vi "Voltage Logging.vi"() -> ()   [LabVIEW 2014]
uses:
  States.ctl
  <vilib>/Utility/miscctls.llb/LVForegroundBackgroundColorsTypeDef.ctl
  <vilib>/DAQmx/read.llb/DAQmx Read (Analog 1D Wfm NChan 1Samp).vi
  <vilib>/DAQmx/miscellaneous.llb/DAQmx Fill In Error Info.vi
  <vilib>/DAQmx/create/channels.llb/DAQmx Create Channel (AI-Voltage-Basic).vi
panel:
  out "Timer":dbl format="%#_g sec"
  in  "maximum value":dbl=1.0 format="%#_13g"
  in  "minimum value":dbl=-1.0 format="%#_13g"
  in  "input terminal configuration":i32(ring)=10083 items=["default"=-1, "RSE"=10083, "NRSE"=10078, "Differential"=10106, "Pseudodifferential"=12529]
  in  "Connect":bool
  out "Logging speed calculated":dbl=3.6
  in  "Time format":bool=TRUE
  out "Error messeage":string
  out "Communication with CDaq":bool
  in  "Channels":tag="cDAQ3Mod1/ai0:7, cDAQ3Mod2/ai0:7, cDAQ3Mod3/ai0:7"
  in  "Upper Limit 3":dbl[](array[numeric])=[0.0, 0.0, 0.0, 0.0, 0.0, 0.0, 0.0, 0.0, 1000.0, 1000.0, 1000.0, 1000.0, 1000.0, 1000.0, 1000.0, 1000.0, 1000.0, 1000.0, 1000.0, 1000.0, 1000.0, 1000.0, 1000.0, 1000.0, 1000.0, 1000.0, 1000.0, 1000.0, 1000.0, 1000.0, 1000.0, 1000.0]
  in  "Upper Limit 2":dbl[](array[numeric])=[0.0, 0.0, 0.0, 0.0, 0.0, 0.0, 0.0, 0.0, 1000.0, 1000.0, 1000.0, 1000.0, 1000.0, 1000.0, 1000.0, 1000.0, 1000.0, 1000.0, 1000.0, 1000.0, 1000.0, 1000.0, 1000.0, 1000.0, 1000.0, 1000.0, 1000.0, 1000.0, 1000.0, 1000.0, 1000.0, 1000.0]
  in  "Lower Limit 3":dbl[](array[numeric])=[-400.0, -400.0, -400.0, -400.0, -400.0, -400.0, -400.0, -400.0, -1000.0, -1000.0, -1000.0, -1000.0, -1000.0, -1000.0, -1000.0, -1000.0, -1000.0, -1000.0, -1000.0, -1000.0, -1000.0, -1000.0, -1000.0, -1000.0, -1000.0, -1000.0, -1000.0, -1000.0, -1000.0, -1000.0, -1000.0, -1000.0, -10000.0, -1000.0]
  in  "Lower Limit 2":dbl[](array[numeric])=[-400.0, -400.0, -400.0, -400.0, -400.0, -400.0, -400.0, -400.0, -1000.0, -1000.0, -1000.0, -1000.0, -1000.0, -1000.0, -1000.0, -1000.0, -1000.0, -1000.0, -1000.0, -1000.0, -1000.0, -1000.0, -1000.0, -1000.0, -1000.0, -1000.0, -1000.0, -1000.0, -1000.0, -1000.0, -1000.0, -1000.0, -10000.0, -1000.0]
  in  "Channel Name 3":string[](array[string])=["STDFA-13", "STDFA-14", "STDFA-15", "STDFA-16", "STDFA-17", "STDFA-18", "No", "No", "Sample 2-1", "Sample 2-2", "Sample 2-3", "Sample 2-4", "Sample 2-5", "Sample 2-6", "Sample 2-7", "Sample 2-8", "Sample 3-1", "Sample 3-2", "Sample 3-3", "Sample 3-4", "Sample 3-5", "Sample 3-6", "Sample 3-7", "Sample 3-8", "Channel 25", "Channel 26", "Channel 27", "Channel 28", "Channel 29", "Channel 30", "Channel 31", "Channel 32"]
  in  "Channel Name 2":string[](array[string])=["IND-7", "IND-8", "IND-9", "IND-10", "IND-11", "IND-12", "No", "No", "Sample 2-1", "Sample 2-2", "Sample 2-3", "Sample 2-4", "Sample 2-5", "Sample 2-6", "Sample 2-7", "Sample 2-8", "Sample 3-1", "Sample 3-2", "Sample 3-3", "Sample 3-4", "Sample 3-5", "Sample 3-6", "Sample 3-7", "Sample 3-8", "Channel 25", "Channel 26", "Channel 27", "Channel 28", "Channel 29", "Channel 30", "Channel 31", "Channel 32"]
  out "To Chart":dbl[](array[numeric])=[70.54695373277418, 10.349711390143883, 7.51922355130685, 18.709524383023034, 7.8154373944745705, 12.02825650884127, -6.402827028058501, -31.548091462286674, -93.31739444104286, 3.5496163088758026, 6.22112697925856, 6.715851179669773, 4.506083089902143, 6.484979886054426, 3.747505987517876, -20.0652183361864, -91.63029877543632, -0.5237737702217623, 6.226074724835393, 9.419905426557538, -0.9188868578980165, 8.59675318650909, 7.740674854943624, -15.27466285302956]
  out "Stop":bool=TRUE
  out "In Range?  4":bool[](array[boolean])=[TRUE, TRUE, TRUE, TRUE, TRUE, TRUE, TRUE, TRUE]
  out "In Range?  3":bool[](array[boolean])=[TRUE, TRUE, TRUE, TRUE, TRUE, TRUE, TRUE, TRUE]
  out "In Range?  2":bool[](array[boolean])=[TRUE, TRUE, TRUE, TRUE, TRUE, TRUE, TRUE, TRUE]
  out "SAMPLE 3":dbl[](array[numeric])=[-91.63029877543632, -0.5237737702217623, 6.226074724835393, 9.419905426557538, -0.9188868578980165, 8.59675318650909, 7.740674854943624, -15.27466285302956] format="%#.1f"
  out "SAMPLE 2":dbl[](array[numeric])=[-93.31739444104286, 3.5496163088758026, 6.22112697925856, 6.715851179669773, 4.506083089902143, 6.484979886054426, 3.747505987517876, -20.0652183361864] format="%#.1f"
  out "SAMPLE 1":dbl[](array[numeric])=[70.54695373277418, 10.349711390143883, 7.51922355130685, 18.709524383023034, 7.8154373944745705, 12.02825650884127, -6.402827028058501, -31.548091462286674] format="%#.1f"
  out "CHANNEL 1-8 SAMPLE 3":T1(graph)={"Numeric"=-91.56444653578738, "Numeric"=-0.2932911360215918, "Numeric"=6.489483443591846, "Numeric"=9.716240232547184, "Numeric"=-0.6554781327134408, "Numeric"=8.761383634660817, "Numeric"=7.740674854943624, "Numeric"=-15.406367224861299}
  out "CHANNEL 1-8   SAMPLE 2":T1(graph)={"Numeric"=-92.75670672596173, "Numeric"=3.945395666258387, "Numeric"=6.682869566286414, "Numeric"=6.913740860038615, "Numeric"=4.60502792945394, "Numeric"=6.419016659336254, "Numeric"=3.7145243744040615, "Numeric"=-20.16416317419381}
  in  "Channel Name":string[](array[string])=["LKS-1", "LKS-2", "LKS-3", "LKS-4", "LKS-5", "LKS-6", "No", "No", "Sample 2-1", "Sample 2-2", "Sample 2-3", "Sample 2-4", "Sample 2-5", "Sample 2-6", "Sample 2-7", "Sample 2-8", "Sample 3-1", "Sample 3-2", "Sample 3-3", "Sample 3-4", "Sample 3-5", "Sample 3-6", "Sample 3-7", "Sample 3-8", "Channel 25", "Channel 26", "Channel 27", "Channel 28", "Channel 29", "Channel 30", "Channel 31", "Channel 32"]
  in  "Logging Speed":dbl=0.001 format="%#_g h"
  out "CHANNEL 1-8 SAMPLE 1":T1(graph)={"Numeric"=69.98743853157956, "Numeric"=9.888934299429126, "Numeric"=7.025533812893019, "Numeric"=18.347485234778834, "Numeric"=7.617961499019248, "Numeric"=11.929518560566871, "Numeric"=-6.43573967719425, "Numeric"=-31.44935350980207}
  in  "Lower Limit":dbl[](array[numeric])=[-400.0, -400.0, -400.0, -400.0, -400.0, -400.0, -400.0, -400.0, -1000.0, -1000.0, -1000.0, -1000.0, -1000.0, -1000.0, -1000.0, -1000.0, -1000.0, -1000.0, -1000.0, -1000.0, -1000.0, -1000.0, -1000.0, -1000.0, -1000.0, -1000.0, -1000.0, -1000.0, -1000.0, -1000.0, -1000.0, -1000.0, -10000.0, -1000.0]
  in  "Upper Limit":dbl[](array[numeric])=[0.0, 0.0, 0.0, 0.0, 0.0, 0.0, 0.0, 0.0, 1000.0, 1000.0, 1000.0, 1000.0, 1000.0, 1000.0, 1000.0, 1000.0, 1000.0, 1000.0, 1000.0, 1000.0, 1000.0, 1000.0, 1000.0, 1000.0, 1000.0, 1000.0, 1000.0, 1000.0, 1000.0, 1000.0, 1000.0, 1000.0]
  out "Potential (mV)":dbl[](array[numeric])=[70.54695373277418, 10.349711390143883, 7.51922355130685, 18.709524383023034, 7.8154373944745705, 12.02825650884127, -6.402827028058501, -31.548091462286674, -93.31739444104286, 3.5496163088758026, 6.22112697925856, 6.715851179669773, 4.506083089902143, 6.484979886054426, 3.747505987517876, -20.0652183361864, -91.63029877543632, -0.5237737702217623, 6.226074724835393, 9.419905426557538, -0.9188868578980165, 8.59675318650909, 7.740674854943624, -15.27466285302956] format="%#.1f"
  in  "Start":bool
  in  "Stop":bool
  # "Potential Logging 2015"
  # "Time until next logging point"
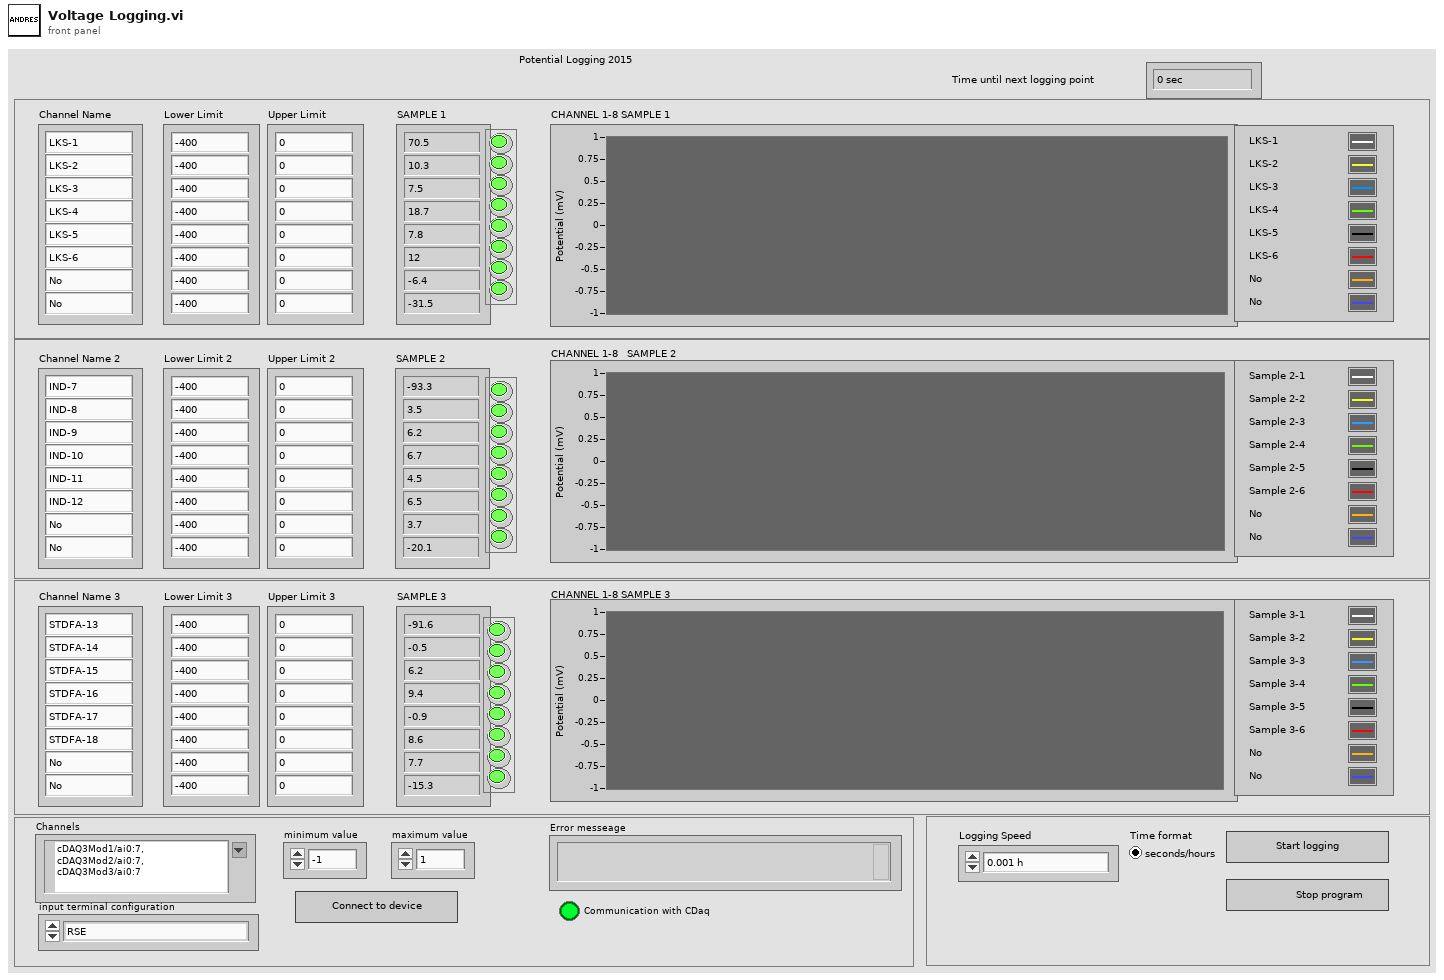
[diagram p1: front panel]
types:
  T1 = cluster{"Numeric":dbl, "Numeric":dbl, "Numeric":dbl, "Numeric":dbl, "Numeric":dbl, "Numeric":dbl, "Numeric":dbl, "Numeric":dbl}
  T2 = typedef "LVForegroundBackgroundColorsTypeDef.ctl" = cluster{"Foreground Color":u32, "Background Color":u32}
  T3 = enum8{"Enabled", "Disabled", "Disabled and Grayed Out"}
  T4 = typedef "States.ctl" = enum16{"Init", "Create File", "Logging", "Stop Program", "Connect"}
  T5 = enum16{"open", "replace", "create", "open or create", "replace or create", "replace or create with confirmation"}
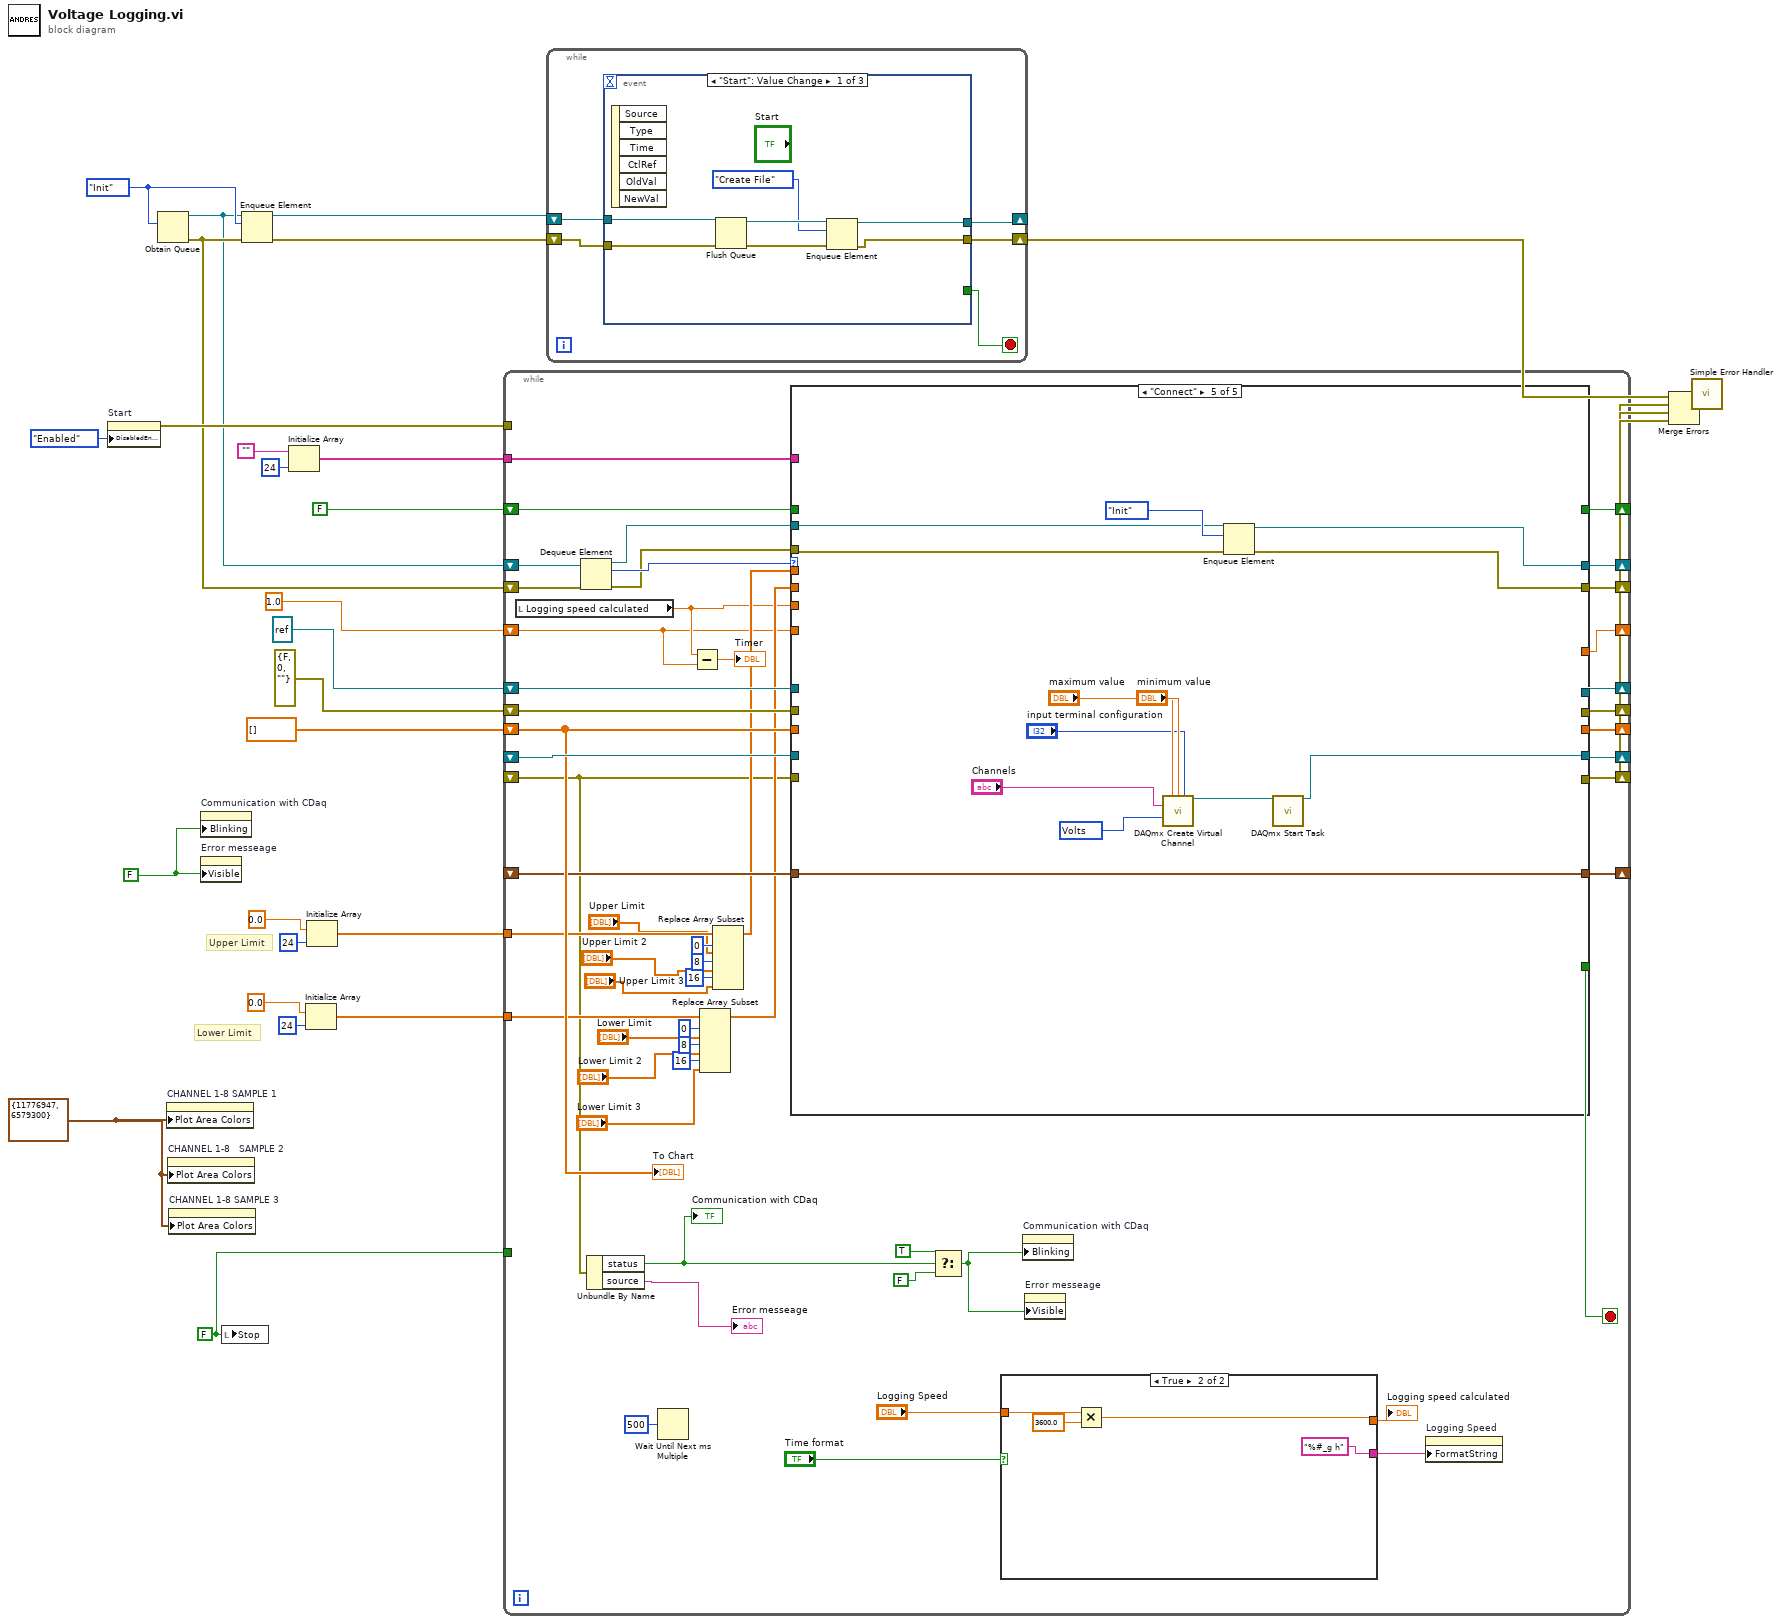
[diagram p0: block diagram]
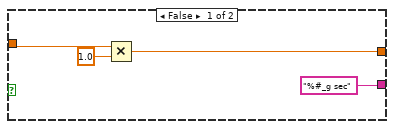
[diagram p2: hidden frame]
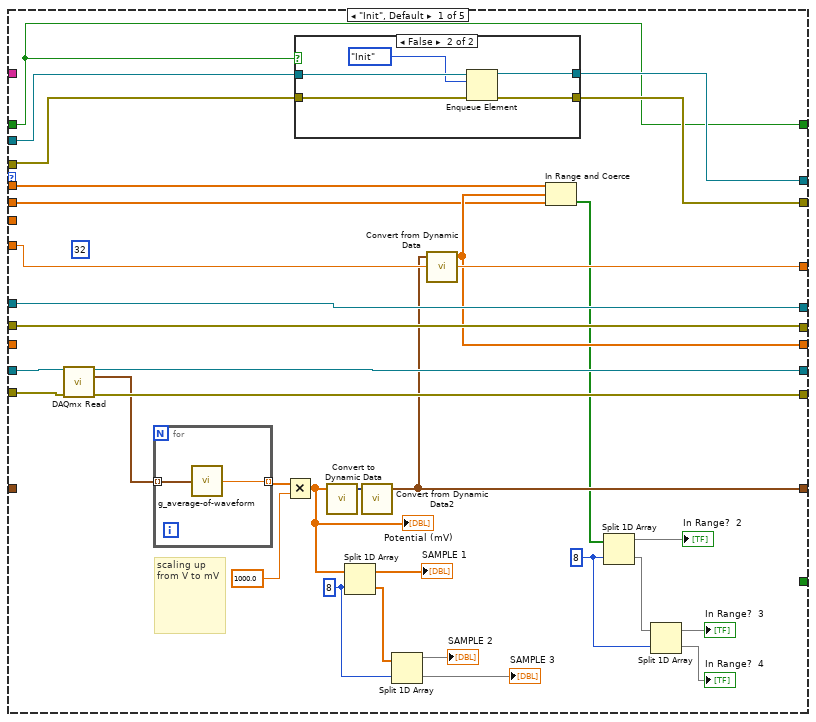
[diagram p3: hidden frame]
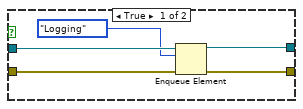
[diagram p4: hidden frame]
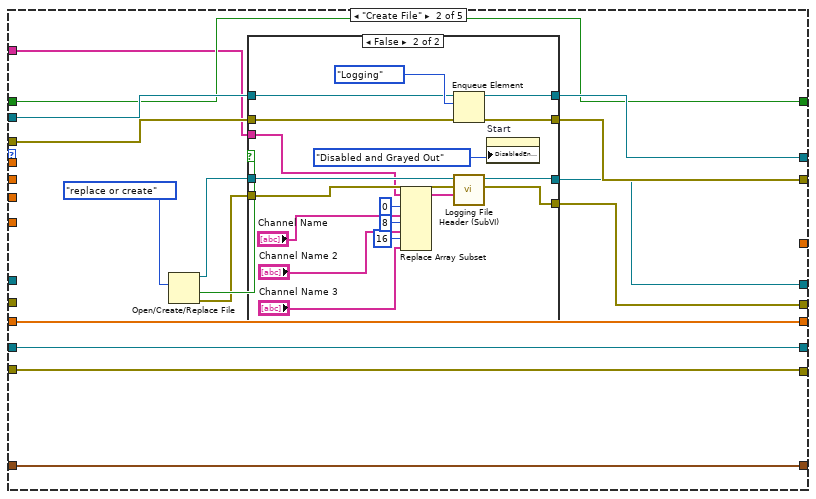
[diagram p5: hidden frame]
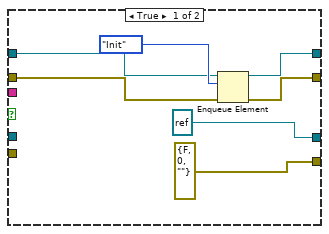
[diagram p6: hidden frame]
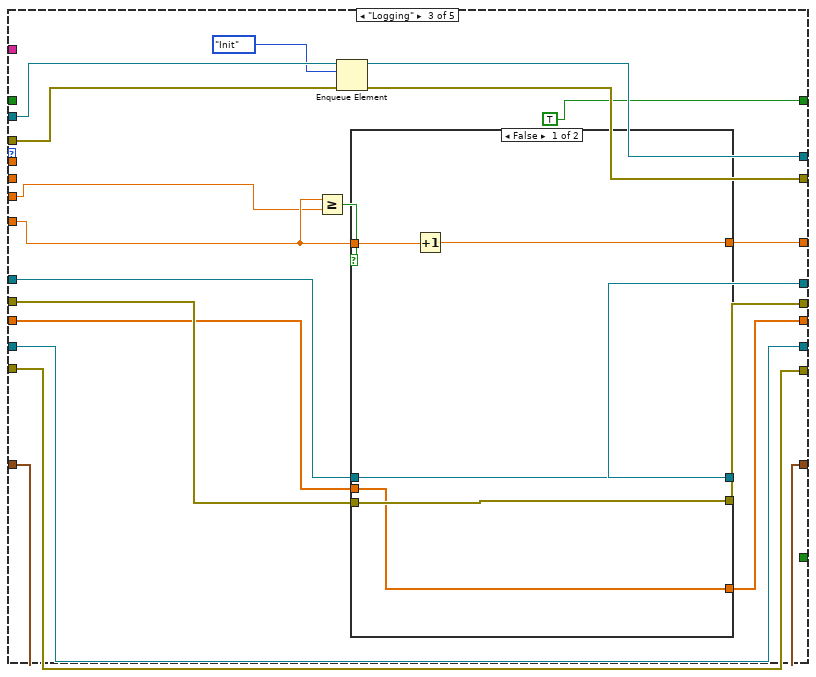
[diagram p7: hidden frame]
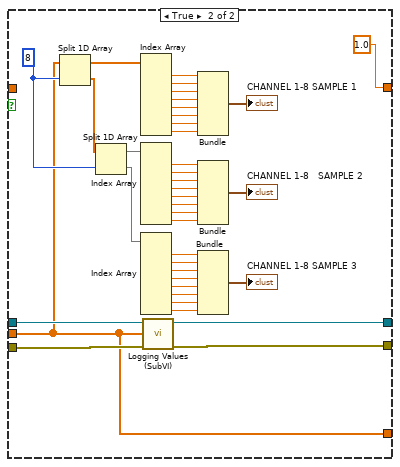
[diagram p8: hidden frame]
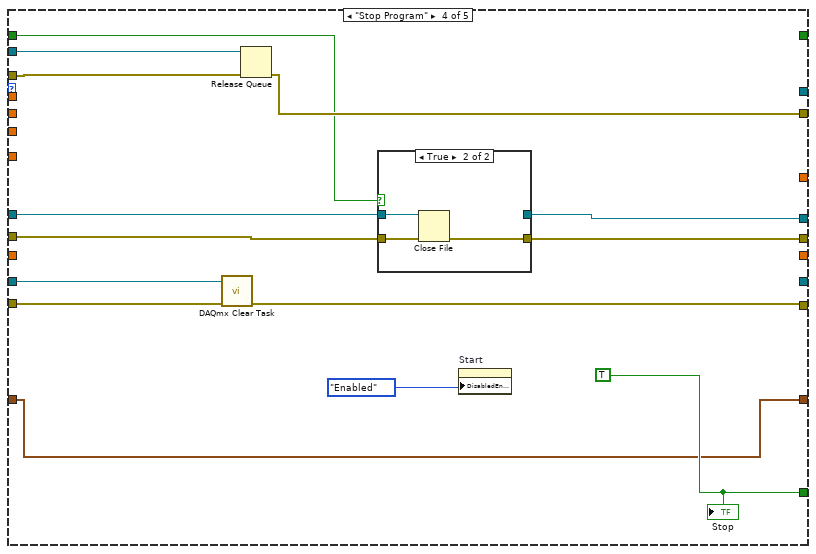
[diagram p9: hidden frame]
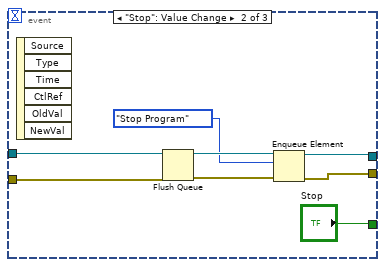
[diagram p11: hidden frame]
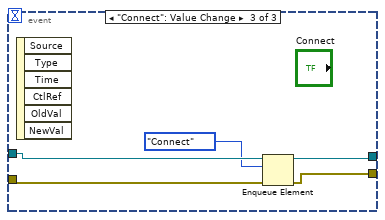
[diagram p12: hidden frame]
diagram:
  w1 = FALSE ("Visible")
  w11 = FALSE ("Stop")
  w12 = T2 {"Foreground Color"=11776947, "Background Color"=6579300} ("Plot Area:Colors 2")
  w27 = States."Init" ("States")
  # "Lower Limit"
  # "Upper Limit"
  n1 = property on="Start" class="Bool"("DisabledEnum"=T3."Enabled" ("Disabled")) -> (error out=w22:errorcluster)  [unwired: 2 in, 1 out]
  n2 = Obtain Queue(element data type=w27) -> (queue out=w19:refnum<queue>, error out=w20:errorcluster)  [unwired: 4 in, 1 out]
  n3 = property on="CHANNEL 1-8 SAMPLE 1" class="WFChart (strict)"("Plot Area Colors"=w12) -> ()  [unwired: 2 in, 2 out]
  n4 = property on="CHANNEL 1-8   SAMPLE 2" class="WFChart (strict)"("Plot Area Colors"=w12) -> ()  [unwired: 2 in, 2 out]
  n5 = property on="CHANNEL 1-8 SAMPLE 3" class="WFChart (strict)"("Plot Area Colors"=w12) -> ()  [unwired: 2 in, 2 out]
  n6 = property on="Communication with CDaq" class="Bool (strict)"("Blinking"=w1) -> ()  [unwired: 2 in, 2 out]
  n7 = property on="Error messeage" class="Str"("Visible"=w1) -> ()  [unwired: 2 in, 2 out]
  n8 = local write "Stop"(w11) -> ()
  n9 = Enqueue Element(queue=w19, element=w27, error in (no error)=w20) -> (queue out=w29:refnum<queue>, error out=w28:errorcluster)  [unwired: 1 in, 1 out]
  n10 = Initialize Array("", 24 ("dimension size")) -> (w8:string[])
  n11 = Initialize Array(0.0, 24 ("dimension size")) -> (w2:dbl[])
  n12 = Initialize Array(0.0, 24 ("dimension size")) -> (w3:dbl[])
  n13 = while {
    shift-right: [w77] -> _
    shift-left: w19 -> [w81]
    shift-right: [w76] -> w13
    shift-left: w20 -> [w82]
    shift-right: [w74] -> w15
    shift-left: _ -> [w42]
    shift-right: [w72] -> _
    shift-left: _ -> [w73]
    shift-right: [w63] -> _
    shift-left: dbl[] [] ("Array") -> [w61]
    shift-right: [w70] -> _
    shift-left: refnum<file> refnum ("refnum out") -> [w71]
    shift-right: [w69] -> w14
    shift-left: errorcluster {"status"=FALSE, "code"=0, "source"=""} ("error out") -> [w68]
    shift-right: [w66] -> _
    shift-left: FALSE -> [w67]
    shift-right: [w64] -> _
    shift-left: 1.0 -> [w31]
    tunnel: w22 -> [_]
    shift-right: [w62] -> _
    shift-left: _ -> [w60]
    tunnel: w11 -> [_]
    tunnel: w8 -> [w59]
    tunnel: w3 -> [w52]
    tunnel: w2 -> [w50]
    stop <- w75 stop-if-true
    n14 = local read "Logging speed calculated"() -> (w32:dbl)
    n15 = Dequeue Element(queue=w81, error in (no error)=w82) -> (queue out=w79:refnum<queue>, element=w80:T4, error out=w78:errorcluster)  [unwired: 1 in, 1 out]
    n16 = Unbundle By Name(w42) -> ("status"=w40:bool, "source"=→"Error messeage":string)
    "Communication with CDaq" <- w40
    n17 = Wait Until Next ms Multiple(millisecond multiple=u32 500) -> ()  [unwired: 1 out]
    n18 = Subtract(x=w32, y=w31) -> (x-y=→"Timer":dbl)
    n19 = Replace Array Subset(array=w50, new element #1="Lower Limit", index #1=0 ("index"), new element #2="Lower Limit 2", index #2=8 ("index"), new element #3="Lower Limit 3", index #3=16 ("index")) -> (w49:dbl[])
    n20 = Replace Array Subset(array=w52, new element #1="Upper Limit", index #1=0 ("index"), new element #2="Upper Limit 2", index #2=8 ("index"), new element #3="Upper Limit 3", index #3=16 ("index")) -> (w51:dbl[])
    n21 = case shown="\"Connect\"" w80 {
      tunnel: w79 -> [w122 w150 w194 w247 w268]
      tunnel: w78 -> [w111 w149 w193 w246 w266]
      tunnel: [w121 w148 w192 _ w267] -> w77
      tunnel: [w120 w147 w191 w245 w265] -> w76
      tunnel: [_ _ _ w242 _] -> w75
      tunnel: w42 -> [w119 w143 w178 w250 _]
      tunnel: w73 -> [w118 w144 w177 w251 _]
      tunnel: [w116 w143 w178 w243 _] -> w74
      tunnel: [w117 w144 w177 _ w258] -> w72
      tunnel: [w106 w145 w180 _ _] -> w63
      tunnel: w61 -> [_ w145 w181 _ _]
      tunnel: w71 -> [w114 _ w186 w249 _]
      tunnel: [w114 w138 w189 w241 _] -> w70
      tunnel: [w113 w137 w188 w244 _] -> w69
      tunnel: w68 -> [w113 _ w185 w248 _]
      tunnel: w67 -> [w115 w142 _ w240 _]
      tunnel: [w115 w142 TRUE _ _] -> w66
      tunnel: w31 -> [w112 _ w182 _ _]
      tunnel: [w112 _ w184 _ _] -> w64
      tunnel: [w105 w136 w179 w238 w257] -> w62
      tunnel: w60 -> [_ w136 w179 w238 w257]
      tunnel: w59 -> [_ w135 _ _ _]
      tunnel: w51 -> [w92 _ _ _ _]
      tunnel: w49 -> [w91 _ _ _ _]
      tunnel: w32 -> [_ _ w176 _ _]
      frame "Init", Default {
        w96 = 8 ("index")
        w104 = 8 ("index")
        (unwired) 32 ("index")
        # "scaling up from V to mV"
        n22 = call-poly <vilib>:"DAQmx Read.vi"("task/channels in"=w118, "error in"=w119) -> ("task out"=w117:refnum<k21>, "data"=w110:waveform(dbl)[], "error out"=w116:errorcluster)  [unwired: 11 in]
        n23 = for {
          tunnel: w110 -> [w124] mode=indexing
          tunnel: [w123] -> w109 mode=indexing
          n24 = call "g_average-of-waveform.vi"("element"=w124) -> ("array average"=w123:dbl)
        }
        n25 = Multiply(x=w109, y=1000.0) -> (x*y=w102:dbl[])
        "Potential (mV)" <- w102
        n26 = case shown="False" w115 {
          tunnel: w122 -> [w129 w134]
          tunnel: w111 -> [w128 w133]
          tunnel: [w127 w132] -> w121
          tunnel: [w126 w131] -> w120
          frame True {
            n27 = Enqueue Element(queue=w129, element=States."Logging" ("States"), error in (no error)=w128) -> (queue out=w127:refnum<queue>, error out=w126:errorcluster)  [unwired: 1 in, 1 out]
          }
          frame False {
            n28 = Enqueue Element(queue=w134, element=States."Init" ("States"), error in (no error)=w133) -> (queue out=w132:refnum<queue>, error out=w131:errorcluster)  [unwired: 1 in, 1 out]
          }
        }
        n29 = call "Convert to Dynamic Data"("Array"=w102) -> ("Dynamic Data Type"=w107:dynamicdata)  [unwired: 3 in]
        n30 = Split 1D Array(array=w102, index=w104) -> (first subarray=→"SAMPLE 1":dbl[], second subarray=w103:dbl[])
        n31 = call "Convert from Dynamic Data2"("Dynamic Data Type"=w107) -> ("Array of Waveform"=w105:waveform(dbl)[])  [unwired: 3 in]
        n32 = Split 1D Array(array=w103, index=w104) -> (first subarray=→"SAMPLE 2":dbl[], second subarray=→"SAMPLE 3":dbl[])
        n33 = call "Convert from Dynamic Data"("Dynamic Data Type"=w105) -> ("Array"=w106:dbl[])  [unwired: 3 in]
        n34 = In Range and Coerce(upper limit=w92, x=w106, lower limit=w91) -> (In Range?=w97:bool[])  [unwired: 1 out]
        n35 = Split 1D Array(array=w97, index=w96) -> (first subarray=→"In Range?  2":bool[], second subarray=w98:bool[])
        n36 = Split 1D Array(array=w98, index=w96) -> (first subarray=→"In Range?  3":bool[], second subarray=→"In Range?  4":bool[])
      }
      frame "Create File" {
        n37 = Open/Create/Replace File(operation (0:open)=T5."replace or create") -> (refnum out=w140:refnum<file>, cancelled=w141:bool, error out=w139:errorcluster)  [unwired: 5 in]
        n38 = case shown="False" w141 {
          tunnel: w150 -> [w156 w174]
          tunnel: w149 -> [w155 w173]
          tunnel: [w154 w172] -> w148
          tunnel: [w153 w171] -> w147
          tunnel: w140 -> [_ w170]
          tunnel: w139 -> [_ w169]
          tunnel: [refnum<file> refnum ("refnum out") w168] -> w138
          tunnel: [errorcluster {"status"=FALSE, "code"=0, "source"=""} ("error out") w167] -> w137
          tunnel: w135 -> [_ w158]
          frame True {
            n39 = Enqueue Element(queue=w156, element=States."Init" ("States"), error in (no error)=w155) -> (queue out=w154:refnum<queue>, error out=w153:errorcluster)  [unwired: 1 in, 1 out]
          }
          frame False {
            n40 = Replace Array Subset(array=w158, new element #1="Channel Name", index #1=0 ("index"), new element #2="Channel Name 2", index #2=8 ("index"), new element #3="Channel Name 3", index #3=16 ("index")) -> (w159:string[])
            n41 = Enqueue Element(queue=w174, element=States."Logging" ("States"), error in (no error)=w173) -> (queue out=w172:refnum<queue>, error out=w171:errorcluster)  [unwired: 1 in, 1 out]
            n42 = call "Logging File Header (SubVI).vi"("Channel Name"=w159, "error out"=w169, "file (use dialog)"=w170) -> ("error out 2"=w167:errorcluster, "refnum out"=w168:refnum<file>)  [unwired: 7 in]
            n43 = property on="Start" class="Bool"("DisabledEnum"=T3."Disabled and Grayed Out" ("Disabled")) -> ()  [unwired: 2 in, 2 out]
          }
        }
      }
      frame "Logging" {
        n44 = Greater Or Equal?(x=w182, y=w176) -> (x >= y?=w183:bool)
        n45 = Enqueue Element(queue=w194, element=States."Init" ("States"), error in (no error)=w193) -> (queue out=w192:refnum<queue>, error out=w191:errorcluster)  [unwired: 1 in, 1 out]
        n46 = case shown="False" w183 {
          tunnel: [w199 w237] -> w189
          tunnel: [w198 w236] -> w188
          tunnel: w181 -> [w195 w202]
          tunnel: w186 -> [w199 w235]
          tunnel: w185 -> [w198 w234]
          tunnel: w182 -> [w197 _]
          tunnel: [w196 1.0] -> w184
          tunnel: [w195 w202] -> w180
          frame False {
            n47 = Increment(x=w197) -> (x+1=w196:dbl)
          }
          frame True {
            w229 = 8 ("index")
            n48 = Split 1D Array(array=w202, index=w229) -> (first subarray=w226:dbl[], second subarray=w230:dbl[])
            n49 = Split 1D Array(array=w230, index=w229) -> (first subarray=w228:dbl[], second subarray=w227:dbl[])
            n50 = Index Array(array=w226) -> (element #1=w225:dbl, element #2=w224:dbl, element #3=w223:dbl, element #4=w222:dbl, element #5=w221:dbl, element #6=w220:dbl, element #7=w219:dbl, element #8=w218:dbl)  [unwired: 8 in]
            n51 = Index Array(array=w228) -> (element #1=w217:dbl, element #2=w215:dbl, element #3=w214:dbl, element #4=w213:dbl, element #5=w212:dbl, element #6=w211:dbl, element #7=w210:dbl, element #8=w209:dbl)  [unwired: 8 in]
            n52 = Index Array(array=w227) -> (element #1=w216:dbl, element #2=w208:dbl, element #3=w207:dbl, element #4=w206:dbl, element #5=w205:dbl, element #6=w204:dbl, element #7=w203:dbl, element #8=w200:dbl)  [unwired: 8 in]
            n53 = call "Logging Values (SubVI).vi"("error in (no error)"=w234, "Array"=w202, "Byte Stream File in"=w235) -> ("error out"=w236:errorcluster, "Byte Stream File out"=w237:refnum<file>)  [unwired: 7 in]
            n54 = Bundle("Numeric"=w225, "Numeric"=w224, "Numeric"=w223, "Numeric"=w222, "Numeric"=w221, "Numeric"=w220, "Numeric"=w219, "Numeric"=w218) -> (→"CHANNEL 1-8 SAMPLE 1":T1)  [unwired: 1 in]
            n55 = Bundle("Numeric"=w217, "Numeric"=w215, "Numeric"=w214, "Numeric"=w213, "Numeric"=w212, "Numeric"=w211, "Numeric"=w210, "Numeric"=w209) -> (→"CHANNEL 1-8   SAMPLE 2":T1)  [unwired: 1 in]
            n56 = Bundle("Numeric"=w216, "Numeric"=w208, "Numeric"=w207, "Numeric"=w206, "Numeric"=w205, "Numeric"=w204, "Numeric"=w203, "Numeric"=w200) -> (→"CHANNEL 1-8 SAMPLE 3":T1)  [unwired: 1 in]
          }
        }
      }
      frame "Stop Program" {
        w242 = TRUE
        n57 = call <vilib>:"DAQmx Clear Task.vi"("task in"=w251, "error in"=w250) -> ("error out"=w243:errorcluster)  [unwired: 13 in]
        n58 = Release Queue(queue=w247, error in (no error)=w246) -> (error out=w245:errorcluster)  [unwired: 1 in, 2 out]
        n59 = case shown="True" w240 {
          tunnel: w249 -> [w253 w256]
          tunnel: w248 -> [w252 w255]
          tunnel: [w252 w254] -> w244
          tunnel: [w253 _] -> w241
          frame False {
          }
          frame True {
            n60 = Close File(refnum=w256, error in=w255) -> (error out=w254:errorcluster)  [unwired: 1 out]
          }
        }
        n61 = property on="Start" class="Bool"("DisabledEnum"=T3."Enabled" ("Disabled")) -> ()  [unwired: 2 in, 2 out]
        "Stop" <- w242
      }
      frame "Connect" {
        w263 = 10348 items=["Volts"=10348, "From Custom Scale"=10065] ("units")
        n62 = call-poly <vilib>:"DAQmx Create Virtual Channel.vi"("maximum value"="maximum value", "minimum value"="minimum value", "input terminal configuration"="input terminal configuration", "physical channels"="Channels", "units"=w263) -> ("task out"=w264:refnum<k21>)  [unwired: 9 in, 1 out]
        n63 = Enqueue Element(queue=w268, element=States."Init" ("States"), error in (no error)=w266) -> (queue out=w267:refnum<queue>, error out=w265:errorcluster)  [unwired: 1 in, 1 out]
        n64 = call <vilib>:"DAQmx Start Task.vi"("task/channels in"=w264) -> ("task out"=w258:refnum<k21>)  [unwired: 13 in, 1 out]
      }
    }
    n65 = Select(t=TRUE ("Visible"), s=w40, f=FALSE ("Visible")) -> (s? t:f=w37:bool)
    n66 = case shown="True" "Time format" {
      tunnel: ["%#_g sec" ("Format String") "%#_g h" ("Format String")] -> w35
      tunnel: "Logging Speed" -> [w85 w89]
      tunnel: [w83 w87] -> w33
      frame False {
        n67 = Multiply(x=w85, y=1.0) -> (x*y=w83:dbl)
      }
      frame True {
        n68 = Multiply(x=w89, y=3600.0) -> (x*y=w87:dbl)
      }
    }
    "Logging speed calculated" <- w33
    n69 = property on="Communication with CDaq" class="Bool (strict)"("Blinking"=w37) -> ()  [unwired: 2 in, 2 out]
    n70 = property on="Error messeage" class="Str"("Visible"=w37) -> ()  [unwired: 2 in, 2 out]
    n71 = property on="Logging Speed" class="DigNum (strict)"("FormatString"=w35) -> ()  [unwired: 2 in, 2 out]
    "To Chart" <- w61
  }
  n72 = while {
    shift-right: [w272] -> _
    shift-left: w29 -> [w274]
    shift-right: [w271] -> w26
    shift-left: w28 -> [w273]
    stop <- w270 stop-if-true
    n73 = event shown="[0] \"Start\": Value Change" {
      selector: _ -> [_ _ _]
      dyn-events: _ -> [_ _ _]
      timeout: _ -> [_ _ _]
      tunnel: w274 -> [w279 w285 w293]
      tunnel: w273 -> [w278 w284 w291]
      tunnel: [w277 w287 w294] -> w272
      tunnel: [w276 w286 w290] -> w271
      tunnel: [_ "Stop" _] -> w270
      event "Start": Value Change {
        n74 = event-data() -> ()  [unwired: 1 in, 6 out]
        n75 = Flush Queue(queue=w279, error in (no error)=w278) -> (queue out=w280:refnum<queue>, error out=w281:errorcluster)  [unwired: 1 out]
        n76 = Enqueue Element(queue=w280, element=States."Create File" ("States"), error in (no error)=w281) -> (queue out=w277:refnum<queue>, error out=w276:errorcluster)  [unwired: 1 in, 1 out]
      }
      event "Stop": Value Change {
        n77 = event-data() -> ()  [unwired: 1 in, 6 out]
        n78 = Flush Queue(queue=w285, error in (no error)=w284) -> (queue out=w288:refnum<queue>, error out=w289:errorcluster)  [unwired: 1 out]
        n79 = Enqueue Element(queue=w288, element=States."Stop Program" ("States"), error in (no error)=w289) -> (queue out=w287:refnum<queue>, error out=w286:errorcluster)  [unwired: 1 in, 1 out]
      }
      event "Connect": Value Change {
        n80 = event-data() -> ()  [unwired: 1 in, 6 out]
        n81 = Enqueue Element(queue=w293, element=States."Connect" ("States"), error in (no error)=w291) -> (queue out=w294:refnum<queue>, error out=w290:errorcluster)  [unwired: 1 in, 1 out]
      }
    }
  }
  n82 = Merge Errors(w26, w13, w14, w15) -> (w25:errorcluster)
  n83 = call <vilib>:"Simple Error Handler.vi"("error in (no error)"=w25) -> ()  [unwired: 4 in, 5 out]
